vi "GetColor.vi"(8 "error in (no error)":errorcluster, 11 "ColorGrayScale in":refnum<class "ColorGrayScale.lvclass">) -> (0 "error out":errorcluster, 2 "Color":u32(colorbox), 3 "ColorGrayScale out":refnum<class "ColorGrayScale.lvclass">)   [LabVIEW 2021, in "Picture2D.lvlib" / "ColorGrayScale.lvclass"]
uses:
  ColorGrayScale.lvclass
  Color/Color.lvclass
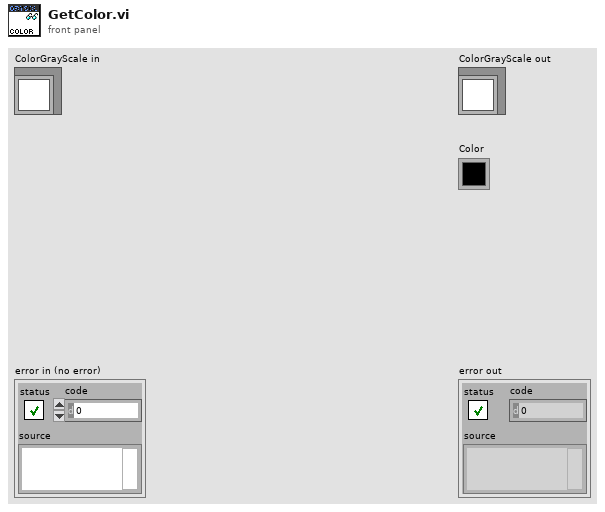
[diagram p1: front panel]
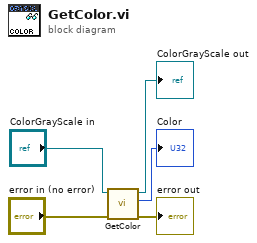
[diagram p0: block diagram]
diagram:
  n1 = call-parent "GetColor.vi"("error in (no error)"="error in (no error)", "Color in"="ColorGrayScale in") -> ("error out"=→"error out":errorcluster, "Color"=→"Color":u32, "Color out"=→"ColorGrayScale out":refnum<class "ColorGrayScale.lvclass">)  [unwired: 7 in]
